vi "Preset.vi"(8 "error in (no error)":errorcluster, 11 "VISA resource name":refnum<visa-resource-name>) -> (0 "error out":errorcluster, 3 "VISA resource name out":refnum<visa-resource-name>)   [LabVIEW 2016, in "Keithley 6517.lvlib"]
doc: "Presets the Keithley Electrometer. This VI also disables continuous scans and aborts any scan in progress. This is included in this VI in part because the unit often tries to treat the \"preset\" commands as triggers if a scan is in progress."
uses:
  <instrlib>/Keithley 6517/Keithley 6517.lvlib
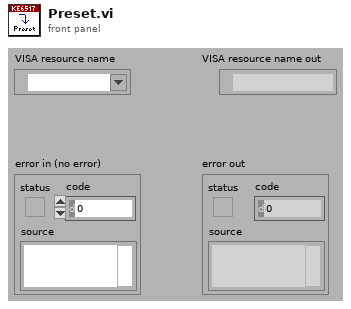
[diagram p1: front panel]
types:
  T1 = typedef "Keithley 6517.lvlib/Extended User Data.ctl" = cluster{"Instrument Model":i32}
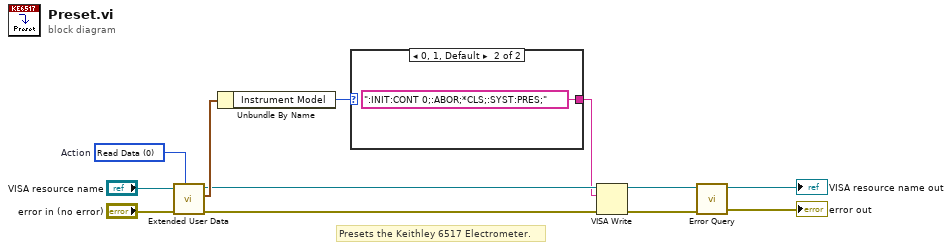
[diagram p0: block diagram]
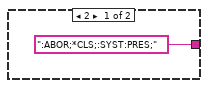
[diagram p2: hidden frame]
diagram:
  w6 = u16 0 items=["Read Data", "Write Data", "Clear Data", "Clear ALL Data"]  # Action
  # "Presets the Keithley 6517 Electrometer."
  n1 = call <instrlib>:"Extended User Data.vi"("Action (0: Read Data)"=w6, "error in (no error)"="error in (no error)", "VISA resource name"="VISA resource name") -> ("error out"=w3:errorcluster, "User Data Out"=w5:T1, "VISA resource name out"=w2:refnum<visa-resource-name>)  [unwired: 6 in]
  n2 = Unbundle By Name(w5) -> ("Instrument Model"=w4:i32)
  n3 = case shown="0, 1, Default" w4 {
    tunnel: [":ABOR;*CLS;:SYST:PRES;" ":INIT:CONT 0;:ABOR;*CLS;:SYST:PRES;"] -> w1
    frame 2 {
    }
    frame 0, 1, Default {
    }
  }
  n4 = VISA Write(VISA resource name=w2, write buffer=w1, error in (no error)=w3) -> (VISA resource name out=w12:refnum<visa-resource-name>, error out=w11:errorcluster)  [unwired: 1 out]
  n5 = call <instrlib>:"Error Query.vi"("error in (no error)"=w11, "VISA resource name"=w12) -> ("error out"=→"error out":errorcluster, "VISA resource name out"=→"VISA resource name out":refnum<visa-resource-name>)  [unwired: 6 in, 2 out]
